vi "essai.vi"() -> ()   [LabVIEW 2015]
panel:
  out "reshape array":i32[][](array[numeric])
  out "subarray 6":i32[](array[numeric])
  out "subarray 5":i32[](array[numeric])
  out "subarray 4":i32[](array[numeric])
  out "appended array":i32[](array[numeric])
  out "interleaved array":i32[](array[numeric])
  out "subarray 3":i32[](array[numeric])
  out "subarray 2":i32[](array[numeric])
  out "subarray":i32[](array[numeric])
  out "Array":i32[][](array[numeric])
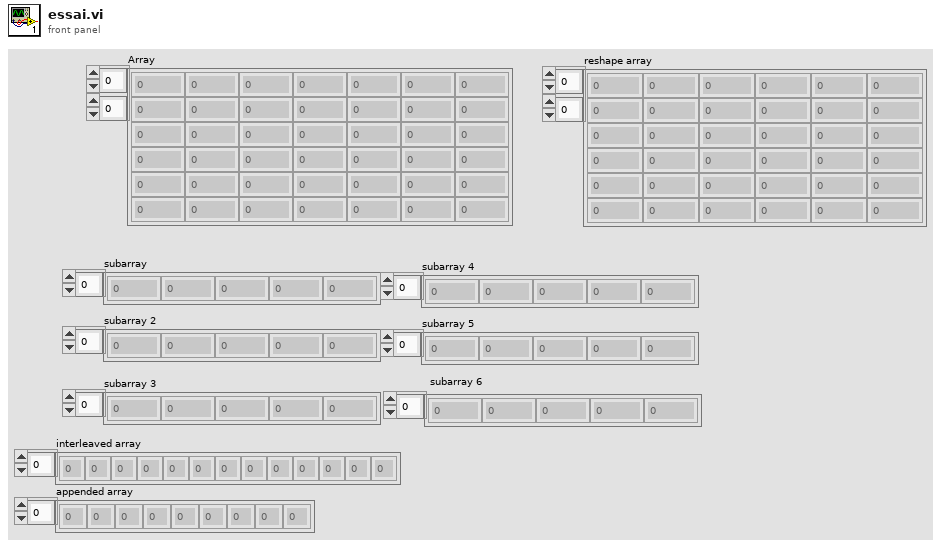
[diagram p1: front panel]
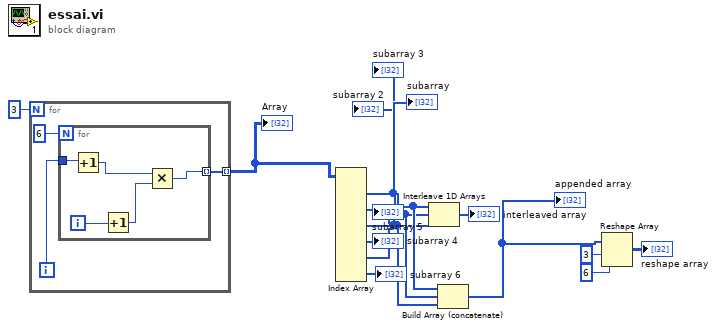
[diagram p0: block diagram]
diagram:
  n1 = for {
    N: 3 -> [_]
    tunnel: [w14] -> w12 mode=indexing
    i -> [w16]
    n2 = for {
      N: 6 -> [_]
      tunnel: w16 -> [w20]
      tunnel: [w21] -> w14 mode=indexing
      i -> [w19]
      n3 = Increment(x=w20) -> (x+1=w18:i32)
      n4 = Increment(x=w19) -> (x+1=w17:i32)
      n5 = Multiply(x=w18, y=w17) -> (x*y=w21:i32)
    }
  }
  "Array" <- w12
  n6 = Index Array(array=w12) -> (element #1=w10:i32[], element #2=w9:i32[], element #3=w8:i32[], element #4=→"subarray 4":i32[], element #5=→"subarray 5":i32[], element #6=→"subarray 6":i32[])  [unwired: 12 in]
  "subarray" <- w10
  "subarray 2" <- w9
  "subarray 3" <- w8
  n7 = Interleave 1D Arrays(w10, w9, w8) -> (→"interleaved array":i32[])
  n8 = Build Array (concatenate)(w10, w9, w8) -> (w4:i32[])
  "appended array" <- w4
  n9 = Reshape Array(w4, 3 ("dimension size"), 6 ("dimension size")) -> (→"reshape array":i32[][])
